vi "Read from File.vi"(8 "error in (no error)":errorcluster, 10 "INI Ref":T1, 11 "Keyboard Macro in":refnum<class "Keyboard Macro.lvclass">) -> (0 "error out":errorcluster, 2 "INI Ref out":T1, 3 "Keyboard Macro out":refnum<class "Keyboard Macro.lvclass">)   [LabVIEW 2020, in "MacroAssert.lvlib" / "Keyboard Macro.lvclass"]
uses:
  Keyboard Macro.lvclass
  C:/Users/acasalen/Documents/LabVIEW Data/Projects/MacroAssert/source/Classes/Step/Step.lvclass
  Macro Step/Macro Step.lvclass
  <vilib>/Utility/config.llb/NI_LVConfig.lvlib
  MacroAssert.lvlib
  <vilib>/Utility/config.llb/Read Key (Boolean).vi
  <vilib>/Utility/config.llb/Read Key (I32).vi
  <vilib>/Utility/config.llb/Config Data RefNum.ctl
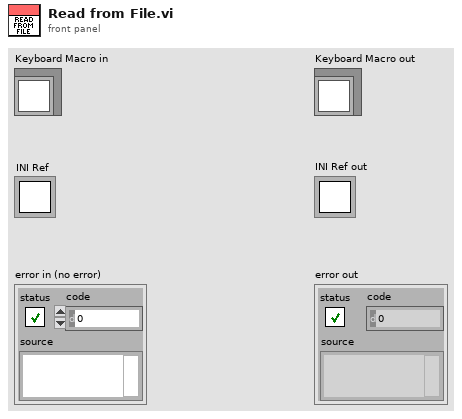
[diagram p1: front panel]
types:
  T1 = typedef "NI_LVConfig.lvlib/Config Data RefNum.ctl" = refnum<k1>
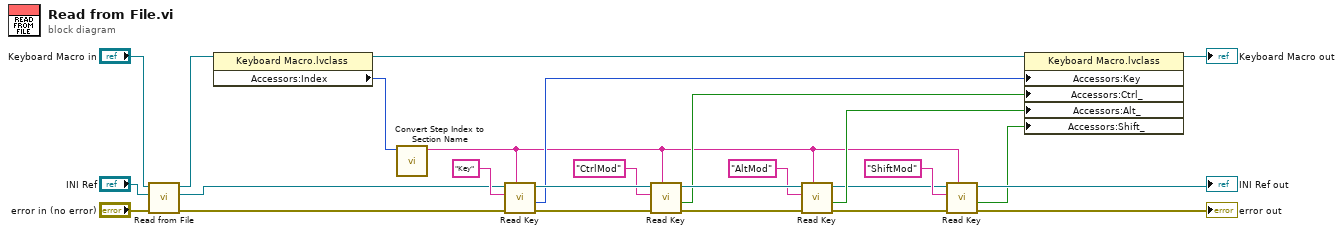
[diagram p0: block diagram]
diagram:
  n1 = call-parent "Read from File.vi"("error in (no error)"="error in (no error)", "INI Ref"="INI Ref", "Step in"="Keyboard Macro in") -> ("error out"=w11:errorcluster, "INI Ref out"=w1:T1, "Step out"=w10:refnum<class "Keyboard Macro.lvclass">)  [unwired: 6 in]
  n2 = property class="Keyboard Macro.lvclass"(reference=w10) -> (reference out=w13:refnum<class "Keyboard Macro.lvclass">, "Accessors:Index"=w12:i32)  [unwired: 1 in, 1 out]
  n3 = call "Convert Step Index to Section Name.vi"("Step Index"=w12) -> ("Section Name"=w7:string)  [unwired: 10 in]
  n4 = call-poly <vilib>:"Read Key.vi"("section"=w7, "error in (no error)"=w11, "key"="Key", "refnum"=w1) -> ("error out"=w22:errorcluster, "value"=w18:i32, "refnum out"=w21:T1)  [unwired: 4 in, 1 out]
  n5 = call-poly <vilib>:"Read Key.vi"("section"=w7, "error in (no error)"=w22, "key"="CtrlMod", "refnum"=w21) -> ("error out"=w16:errorcluster, "value"=w15:bool, "refnum out"=w23:T1)  [unwired: 4 in, 1 out]
  n6 = call-poly <vilib>:"Read Key.vi"("section"=w7, "error in (no error)"=w16, "key"="AltMod", "refnum"=w23) -> ("error out"=w8:errorcluster, "value"=w14:bool, "refnum out"=w3:T1)  [unwired: 4 in, 1 out]
  n7 = call-poly <vilib>:"Read Key.vi"("section"=w7, "error in (no error)"=w8, "key"="ShiftMod", "refnum"=w3) -> ("error out"=→"error out":errorcluster, "value"=w2:bool, "refnum out"=→"INI Ref out":T1)  [unwired: 4 in, 1 out]
  n8 = property class="Keyboard Macro.lvclass"(reference=w13, "Accessors:Key"=w18, "Accessors:Ctrl_"=w15, "Accessors:Alt_"=w14, "Accessors:Shift_"=w2) -> (reference out=→"Keyboard Macro out":refnum<class "Keyboard Macro.lvclass">)  [unwired: 1 in, 1 out]
